vi "set_position.vi"(0 "PI_Piezo (in)":refnum<class "PI_Piezo.lvclass">, 11 "error in":errorcluster) -> (4 "PI_Piezo":refnum<class "PI_Piezo.lvclass">, 15 "error out":errorcluster)   [LabVIEW 2013, in "PI_Piezo.lvclass"]
doc: "This VI demonstrates how to initialize an E-816 system with more than one axis, how to move all connected axes and how to query for the position value. \n\nIn this example the E-816 is connected through USB. The Serial No. of the system to command is not known, so the \"Search for controllers\" control is left TRUE. The VI runs E816_Configuration_Setup.vi with specified settings, moves the connected axes relative to their current position, waits for the movement to finish and reads the position of the axes and the error status of the controller. Instead of calling the corresponding command VIs, it uses \"Split multiple axes command.vi\" which sends the chosen commands for the given axes one after another and returns the answer array (if any). The diagram shows how to combine the driver VIs for these tasks. \n\nFor an example of how to command a single axis E-816 system connected through RS-232 see E816_Sample_ Application_1.vi\n\nWarning: Before running this VI, modify the interface settings on the block diagram to reflect your configuration. The predefined settings provided with the VI probably do not match your system."
uses:
  PI_Piezo.lvclass
  PI_Piezo.lvclass/PI_Piezo.ctl
  Experiment/Globals.vi
panel:
  out "Numeric":i32
  # "This VI demonstrates how to initialize an E-816 system with more than one axis, how to move all connected axes and how to query\nfor the position value. The VI runs E816_Configuration_Setup.vi with specified settings, moves the connected axes relative to their \ncurrent position and reads the position. Instead of calling the corresponding command VIs, it uses \"Split multiple axes command.vi\"\nwhich sends the chosen commands for the given axes one after another and returns the answer array (if any). The diagram shows\nhow to combine the driver VIs for these tasks. \n\nWarning: Before running this VI, modify the interface settings on the block diagram to reflect your configuration. The predefined \n                 settings provided with the VI probably do not match your system."
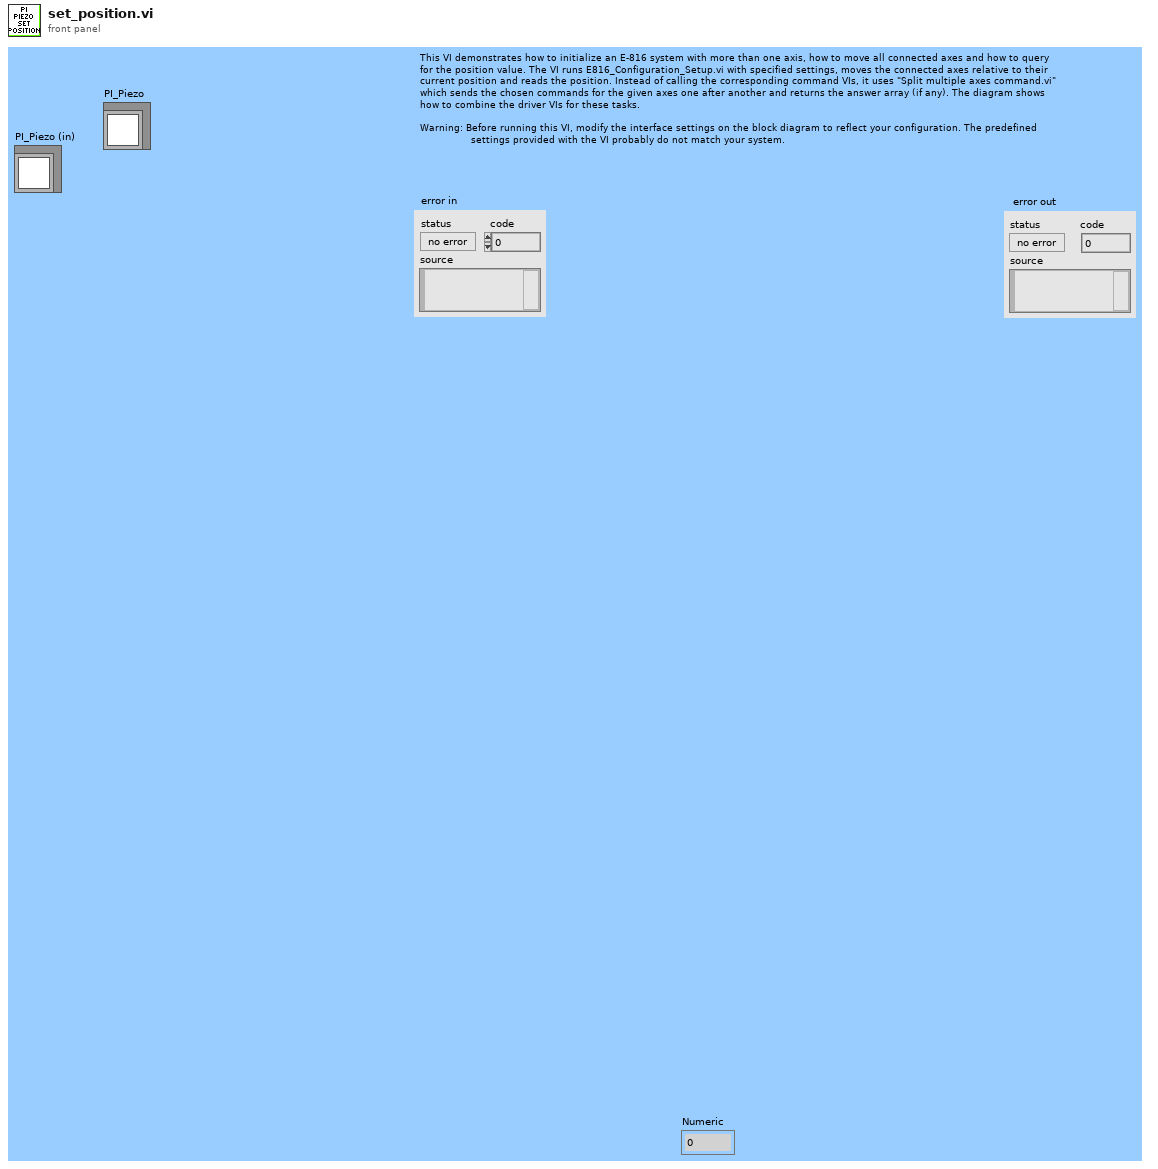
[diagram p1: front panel]
types:
  T1 = enum16{"DCO", "DCO?", "MOV", "MOV?", "MVR", "ONT?", "OVF?", "POS?", "RST", "SVA", "SVA?", "SVO", "SVO?", "SVR", "VOL?", "GWait"}
  T2 = typedef "PI_Piezo.lvclass/settings.ctl" = cluster{"Enable":bool, "Array of Piezo Controllers":T3[]}
  T3 = typedef "PI_Piezo.lvclass/piezo_controller.ctl" = cluster{"Enable":bool, "Serial No.":string, "Array of Piezo Channels":T4[]}
  T4 = typedef "PI_Piezo.lvclass/piezo_channel.ctl" = cluster{"Servo":bool, "Set Position":dbl}
  T5 = cluster{"Axis":string, "Servo":bool, "Position":dbl}
  T6 = cluster{"Identification":string, string, cluster{"Axis":string, "Servo":bool, "Position":dbl}[]}
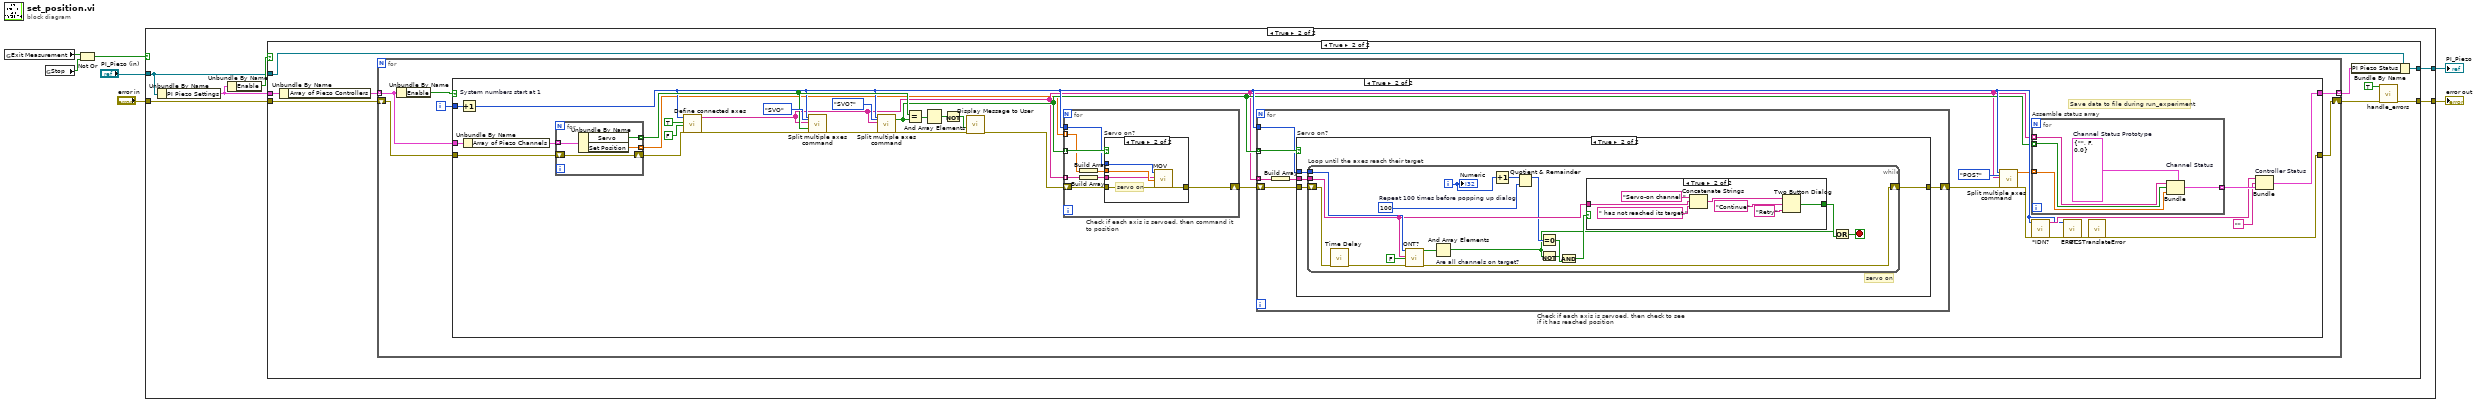
[diagram p0: block diagram]
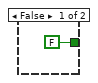
[diagram p6: hidden frame]
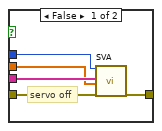
[diagram p7: hidden frame]
diagram:
  n1 = global read "Globals.vi" "Exit Measurement"() -> (w3:bool)
  n2 = global read "Globals.vi" "Stop"() -> (w2:bool)
  n3 = Not Or(1:w2, 2:w3) -> (0:w1:bool)
  n4 = case shown="True" w1 {
    tunnel: "error in" -> [w9 w14]
    tunnel: [w8 w12] -> w6
    tunnel: "PI_Piezo (in)" -> [w8 w11]
    tunnel: [w9 w10] -> w4
    frame False {
    }
    frame True {
      n5 = Unbundle By Name(w11) -> ("PI Piezo Settings"=w13:T2)
      n6 = Unbundle By Name(w13) -> ("Enable"=w15:bool)
      n7 = case shown="True" w15 {
        tunnel: w13 -> [_ w26]
        tunnel: w14 -> [w17 w24]
        tunnel: [w17 w18] -> w10
        tunnel: [w16 w23] -> w12
        tunnel: w11 -> [w16 w21]
        frame False {
        }
        frame True {
          n8 = Unbundle By Name(w26) -> ("Array of Piezo Controllers"=w25:T3[])
          n9 = for {
            tunnel: w25 -> [w30] mode=indexing
            shift-right: [w28] -> w19
            shift-left: w24 -> [w29]
            tunnel: [w27] -> w22 mode=indexing
            i -> [w31]
            n10 = Unbundle By Name(w30) -> ("Enable"=w32:bool)
            n11 = case shown="True" w32 {
              tunnel: w31 -> [_ w34]
              tunnel: w30 -> [_ w66]
              tunnel: w29 -> [w33 w38]
              tunnel: [w33 w62] -> w28
              tunnel: [_ w65] -> w27
              frame False {
              }
              frame True {
                # "Save data to file during run_experiment"
                n12 = Increment "System numbers start at 1"(x=w34) -> (x+1=w44:i32)
                n13 = Unbundle By Name(w66) -> ("Array of Piezo Channels"=w64:T4[])
                n14 = for {
                  tunnel: w64 -> [w129] mode=indexing
                  tunnel: [w128] -> w53 mode=indexing
                  tunnel: [w127] -> w39 mode=indexing
                  shift-right: [w126] -> w37
                  shift-left: w38 -> [w126]
                  n15 = Unbundle By Name(w129) -> ("Servo"=w128:bool, "Set Position"=w127:dbl)
                }
                n16 = call "Define connected axes.vi"("System no."=w44, "Read from\ncontroller?"=TRUE ("Read from\ncontroller?"), "Invert\norder?"=FALSE ("Invert\norder?"), "error in"=w37) -> ("Conn. Axes out"=w41:string[], "error out"=w56:errorcluster)  [unwired: 14 in]
                n17 = call "Split multiple axes command.vi"("System no."=w44, "Command"=T1."SVO", "Axes to command"=w41, "Bool. values in"=w53, "error in"=w56) -> ("error out"=w58:errorcluster)  [unwired: 12 in, 2 out]
                n18 = call "Split multiple axes command.vi"("System no."=w44, "Command"=T1."SVO?", "Axes to command"=w41, "error in"=w58) -> ("Bool. values out"=w42:bool[], "error out"=w51:errorcluster)  [unwired: 13 in, 1 out]
                n19 = Equal?(x=w53, y=w42) -> (x = y?=w52:bool[])
                n20 = And Array Elements(Boolean array=w52) -> (logical AND=w50:bool)
                n21 = Not(x=w50) -> (.not. x?=w49:bool)
                n22 = call "Display Message to User"("error in (no error)"=w51, "Enable"=w49) -> ("error out"=w36:errorcluster)  [unwired: 8 in, 1 out]
                n23 = for "Check if each axis is servoed, then command it to position" {
                  tunnel: w41 -> [w103] mode=indexing
                  tunnel: w42 -> [w110] mode=indexing
                  tunnel: w44 -> [w109]
                  tunnel: w39 -> [w105] mode=indexing
                  shift-right: [w107] -> w43
                  shift-left: w36 -> [w108]
                  n24 = Build Array(w105) -> (w104:dbl[])
                  n25 = Build Array(w103) -> (w106:string[])
                  n26 = case "Servo on?" shown="True" w110 {
                    tunnel: w109 -> [w115 w117]
                    tunnel: w108 -> [w114 w119]
                    tunnel: [w113 w116] -> w107
                    tunnel: w106 -> [w112 w118]
                    tunnel: w104 -> [w111 w120]
                    frame False {
                      # "servo off"
                      n27 = call "SVA.vi"("System no."=w115, "Axes to move"=w112, "PZT voltage"=w111, "error in"=w114) -> ("error out"=w113:errorcluster)  [unwired: 15 in]
                    }
                    frame True {
                      # "servo on"
                      n28 = call "MOV.vi"("System no."=w117, "Axes to move"=w118, "Position values"=w120, "error in"=w119) -> ("error out"=w116:errorcluster)  [unwired: 15 in]
                    }
                  }
                }
                n29 = for "Check if each axis is servoed, then check to see if it has reached position" {
                  tunnel: w41 -> [w67] mode=indexing
                  tunnel: w42 -> [w72] mode=indexing
                  tunnel: w44 -> [w71]
                  shift-right: [w69] -> w40
                  shift-left: w43 -> [w70]
                  n30 = Build Array(w67) -> (w68:string[])
                  n31 = case "Servo on?" shown="True" w72 {
                    tunnel: w71 -> [_ w76]
                    tunnel: w70 -> [w73 w74]
                    tunnel: [w73 w75] -> w69
                    tunnel: w68 -> [_ w77]
                    frame False {
                      # "servo off"
                    }
                    frame True {
                      # "servo on"
                      n32 = while "Loop until the axes reach their target" {
                        shift-right: [w86] -> w75
                        shift-left: w74 -> [w88]
                        tunnel: w77 -> [w89]
                        tunnel: w76 -> [w92]
                        i -> [w81]
                        stop <- w94 stop-if-true
                        w85 = 100  # Repeat 100 times before popping up dialog
                        n33 = call "Time Delay"("error in (no error)"=w88) -> ("error out"=w87:errorcluster)  [unwired: 10 in]
                        n34 = call "ONT?.vi"("System no."=w92, "Axes to query"=w89, "All axes?"=FALSE, "error in"=w87) -> ("Axis on target?"=w90:bool[], "error out"=w86:errorcluster)  [unwired: 14 in]
                        n35 = And Array Elements "Are all channels on target?"(Boolean array=w90) -> (logical AND=w79:bool)
                        n36 = Increment(x=w81) -> (x+1=w80:i32)
                        n37 = Quotient & Remainder(x=w80, y=w85) -> (x-y*floor(x/y)=w84:i32)  [unwired: 1 out]
                        n38 = Equal To 0?(x=w84) -> (x = 0?=w83:bool)
                        n39 = Not(x=w79) -> (.not. x?=w78:bool)
                        n40 = And(x=w78, y=w83) -> (x .and. y?=w82:bool)
                        n41 = case shown="True" w82 {
                          tunnel: [FALSE ("T button?") w100] -> w93
                          tunnel: w89 -> [_ w96]
                          frame False {
                          }
                          frame True {
                            n42 = Concatenate Strings("Servo-on channel " ("string"), w96, " has not reached its target." ("message")) -> (w99:string)
                            n43 = Two Button Dialog(message=w99, 1:"Retry" ("F button name (\"Cancel\")"), 2:"Continue" ("T button name (\"OK\")")) -> (T button?=w100:bool)
                          }
                        }
                        n44 = Or(x=w79, y=w93) -> (x .or. y?=w94:bool)
                        "Numeric" <- w81
                      }
                    }
                  }
                }
                n45 = call "Split multiple axes command.vi"("System no."=w44, "Command"=T1."POS?", "Axes to command"=w41, "error in"=w40) -> ("Num. values out"=w35:dbl[], "error out"=w47:errorcluster)  [unwired: 13 in, 1 out]
                n46 = for "Assemble status array" {
                  tunnel: w42 -> [w125] mode=indexing
                  tunnel: w35 -> [w121] mode=indexing
                  tunnel: [w124] -> w61 mode=indexing
                  tunnel: w41 -> [w123] mode=indexing
                  w122 = T5 {"Axis"="", "Servo"=FALSE, "Position"=0.0}  # Channel Status Prototype
                  n47 = Bundle "Channel Status"(cluster=w122, "Axis"=w123, "Servo"=w125, "Position"=w121) -> (w124:T5)
                }
                n48 = call "*IDN?.vi"("System no."=w44, "error in"=w47) -> ("Identification"=w45:string, "error out"=w46:errorcluster)  [unwired: 16 in]
                n49 = call "ERR?.vi"("System no."=w44, "error in"=w46) -> ("error out"=w63:errorcluster)  [unwired: 16 in, 1 out]
                n50 = call "GCSTranslateError.vi"("error in"=w63) -> ("error out"=w62:errorcluster)  [unwired: 16 in, 2 out]
                n51 = Bundle "Controller Status"("Identification"=w45, "", w61) -> (w65:T6)  [unwired: 1 in]
              }
            }
          }
          n52 = Bundle By Name(cluster=w21, "PI Piezo Status"=w22) -> (w23:refnum<class "PI_Piezo.lvclass">)
          n53 = call "handle_errors.vi"("Exit Operation"=TRUE ("Exit Measurement"), "error in (no error)"=w19) -> ("error out"=w18:errorcluster)  [unwired: 13 in]
        }
      }
    }
  }
  "error out" <- w4
  "PI_Piezo" <- w6
